vi "Save Local Images Direct.vi"(2 "Save Images":bool, 3 "Image Pathnames":path[](array[path]), 4 "Camera Names":string[](array[string])) -> (0 "error out":errorcluster, 1 "Filenames out":path[](array[path]))   [LabVIEW 2022 SP3]
uses:
  Camera Server/Globals/CamServer global.vi
  Anemometry Sub Vis/Globals/Meas_global.vi
  Anemometry Sub Vis/Globals/Extra_Commands_Global.vi
  Picture Display Global.vi
  Anemometry Sub Vis/Globals/Trav_pos_global.vi
panel:
  out "Execution:State":T1(ring)
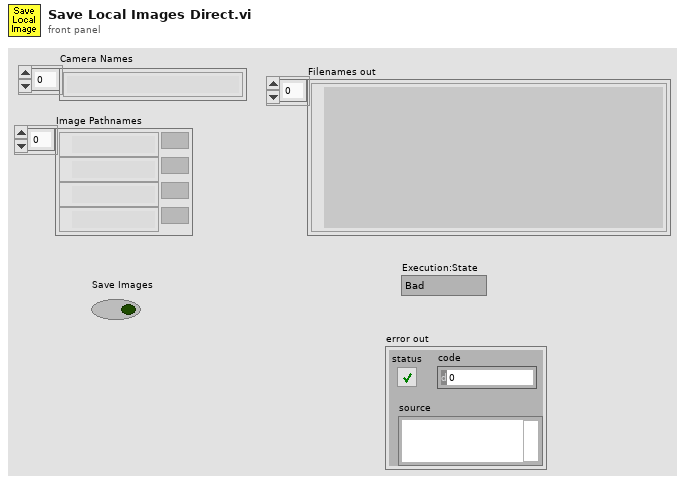
[diagram p1: front panel]
types:
  T1 = enum32{"Bad", "Idle", "Run top level", "Running"}
  T2 = enum32{"Invalid", "Standard", "Closed", "Hidden", "Minimized", "Maximized"}
  T3 = typedef "Camera enum.ctl" = string
  T4 = typedef "IMAQ Image.ctl" = refnum<image>
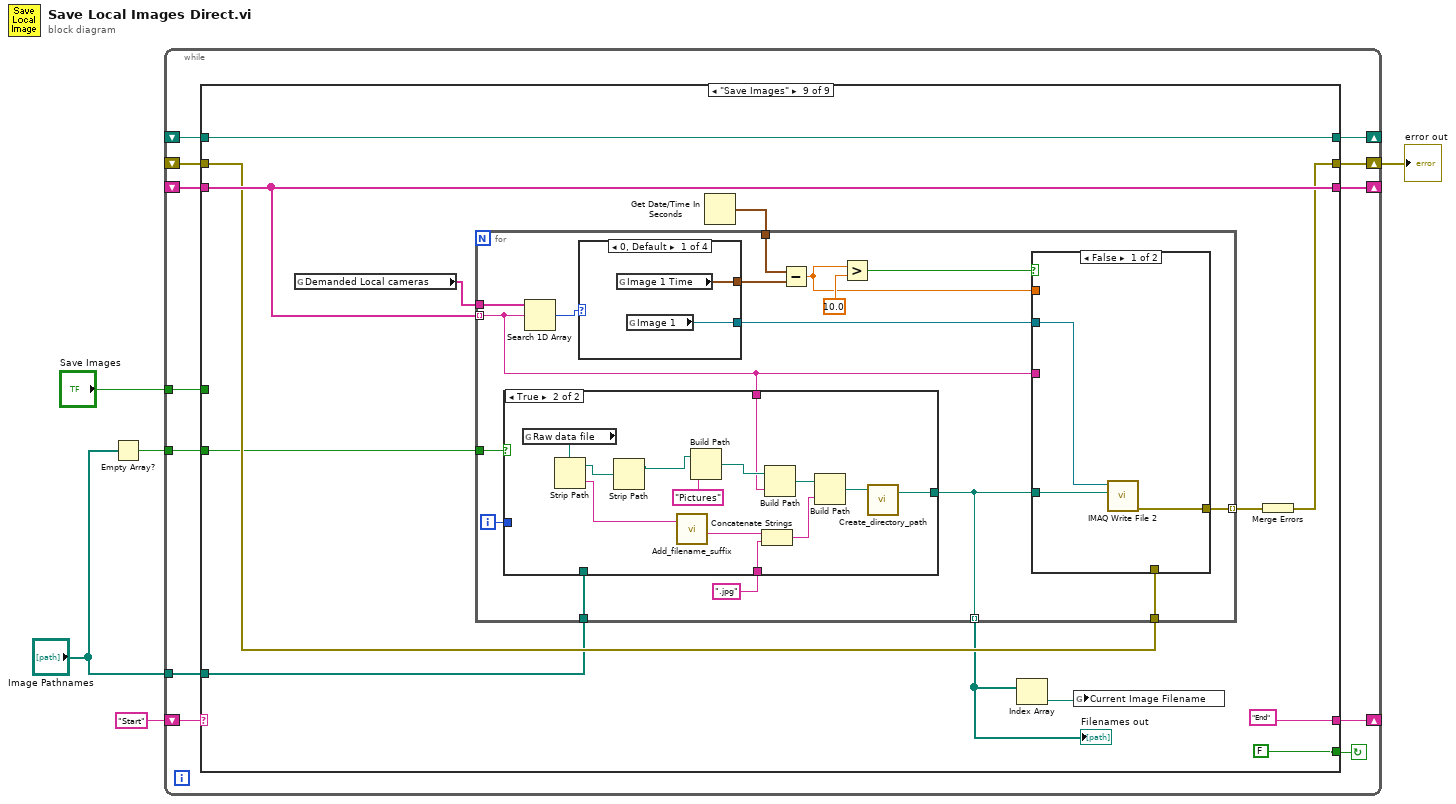
[diagram p0: block diagram]
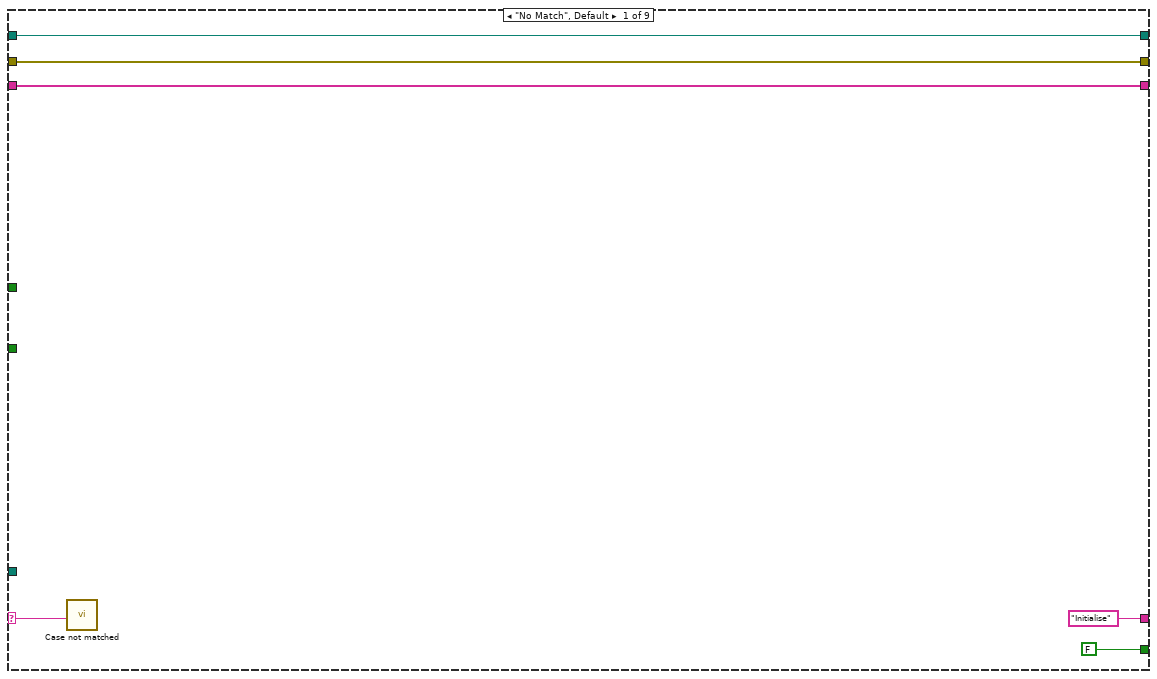
[diagram p2: hidden frame]
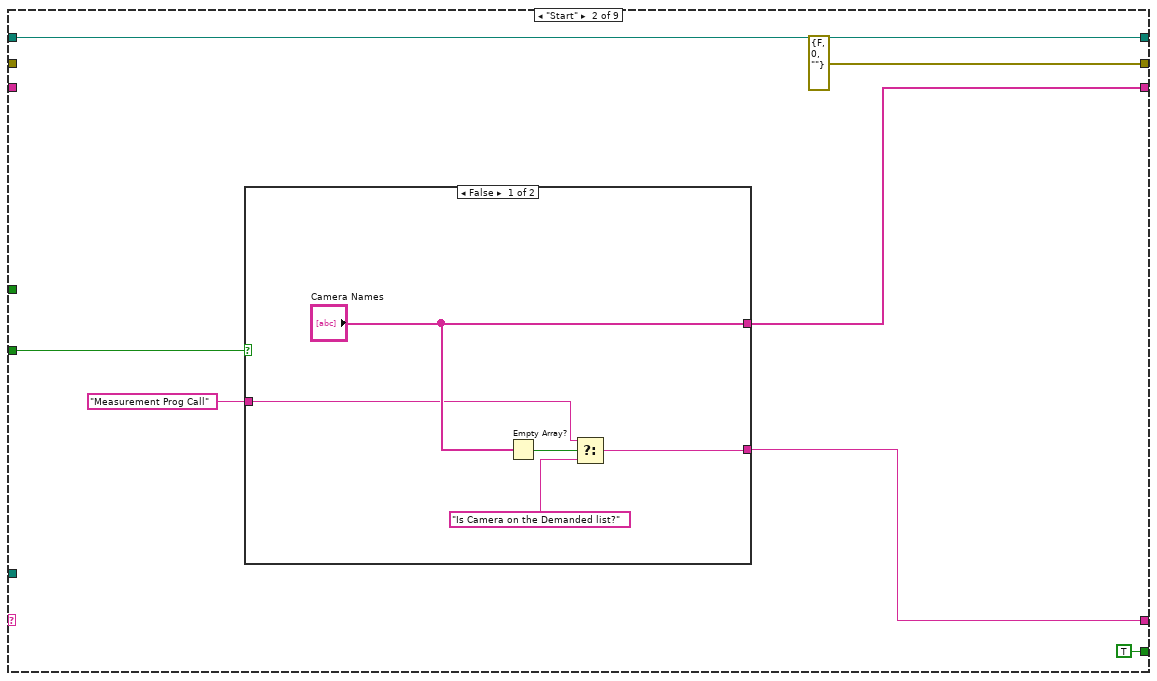
[diagram p3: hidden frame]
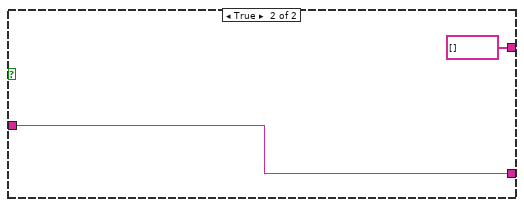
[diagram p4: hidden frame]
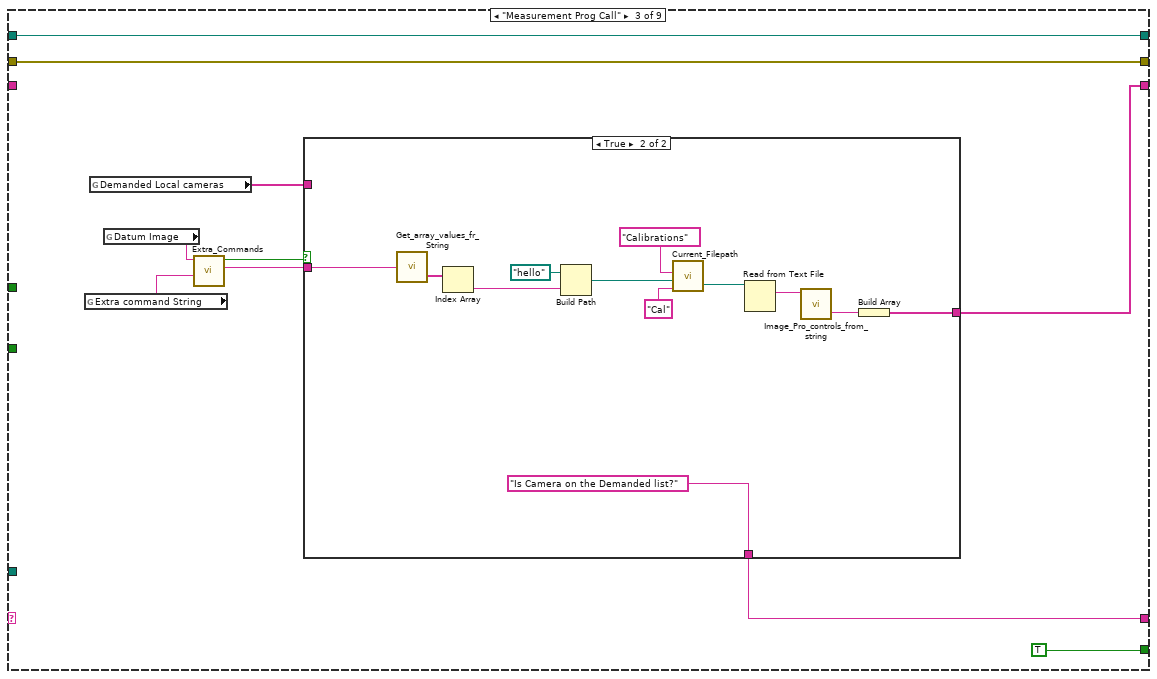
[diagram p5: hidden frame]
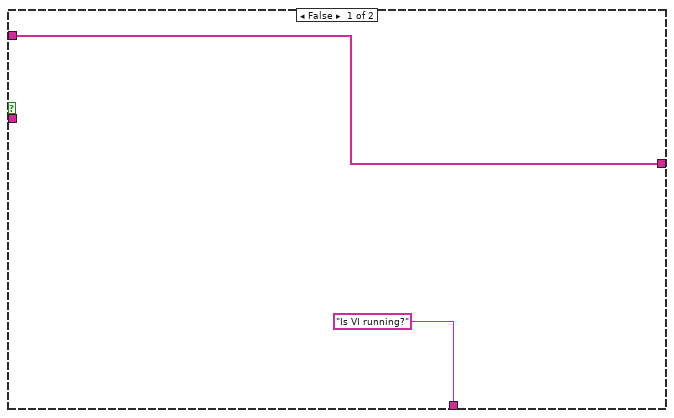
[diagram p6: hidden frame]
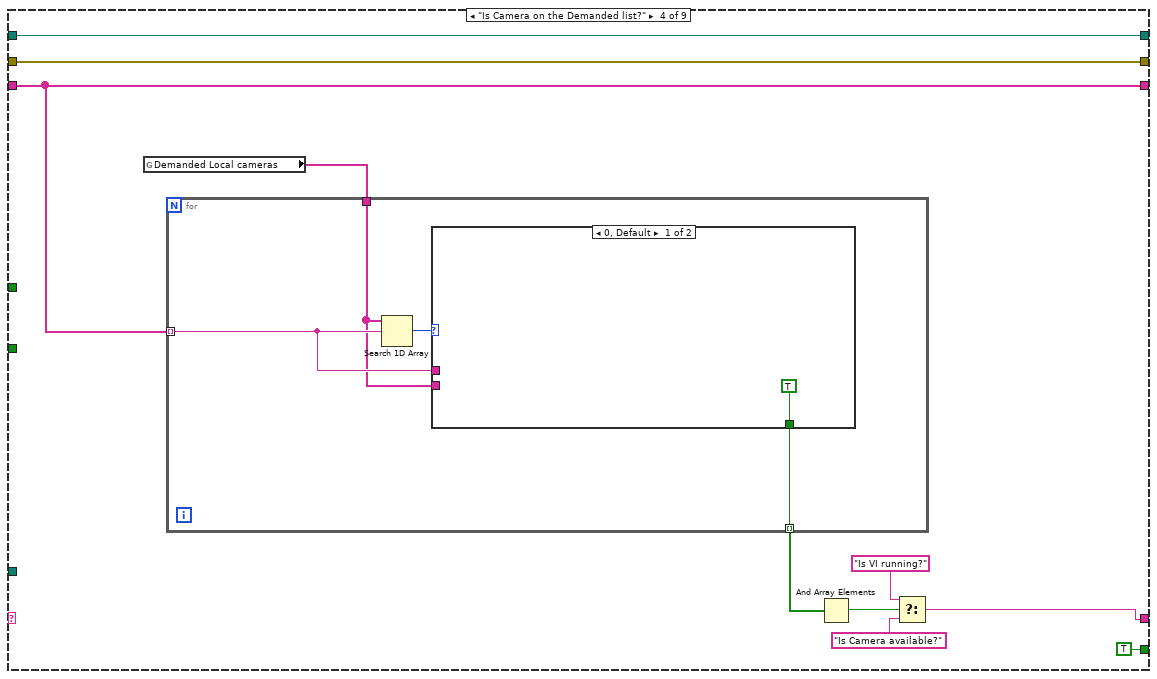
[diagram p7: hidden frame]
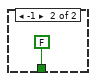
[diagram p8: hidden frame]
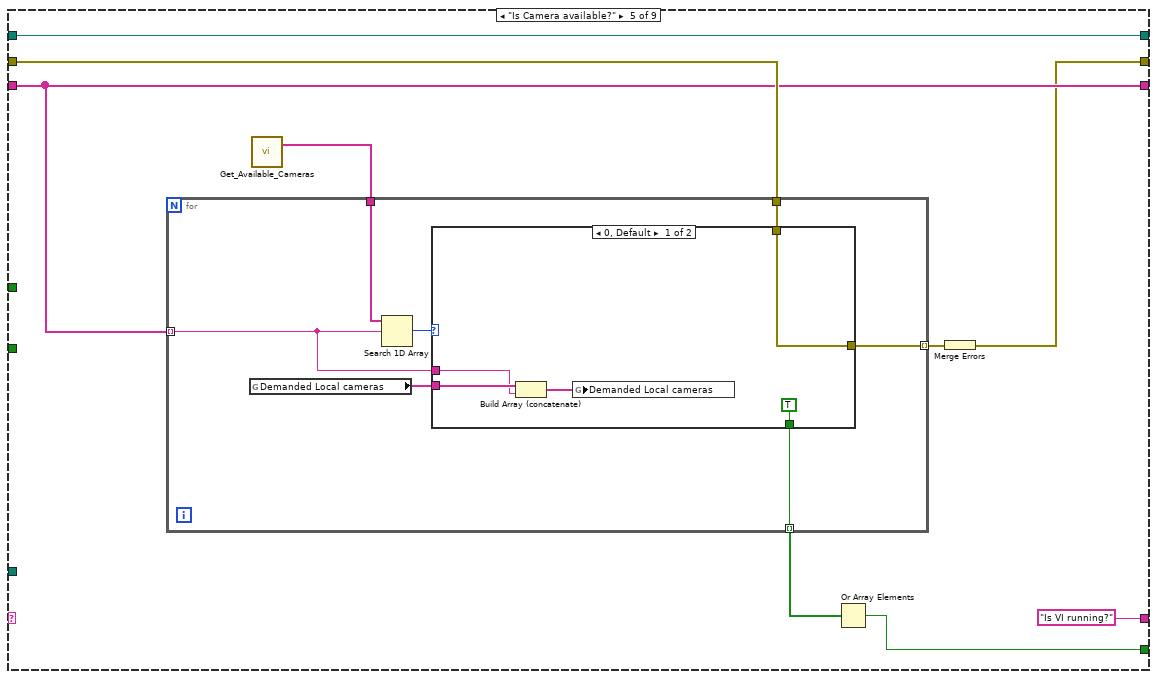
[diagram p9: hidden frame]
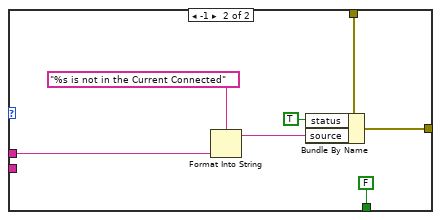
[diagram p10: hidden frame]
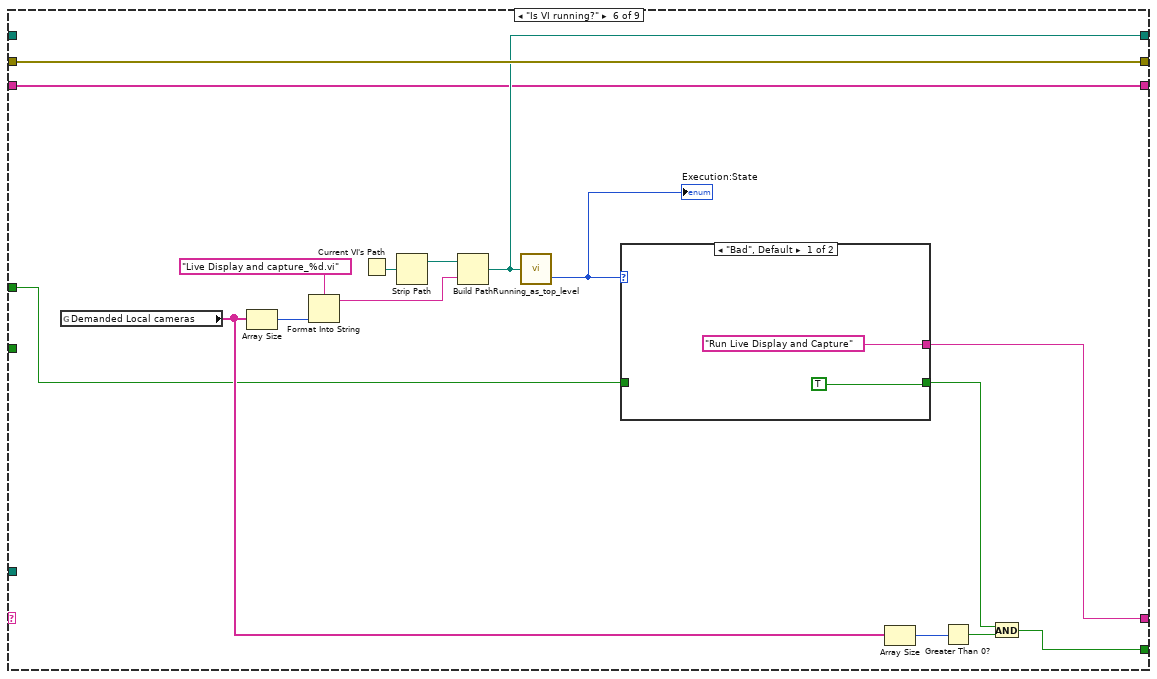
[diagram p11: hidden frame]
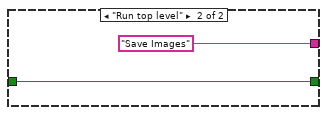
[diagram p12: hidden frame]
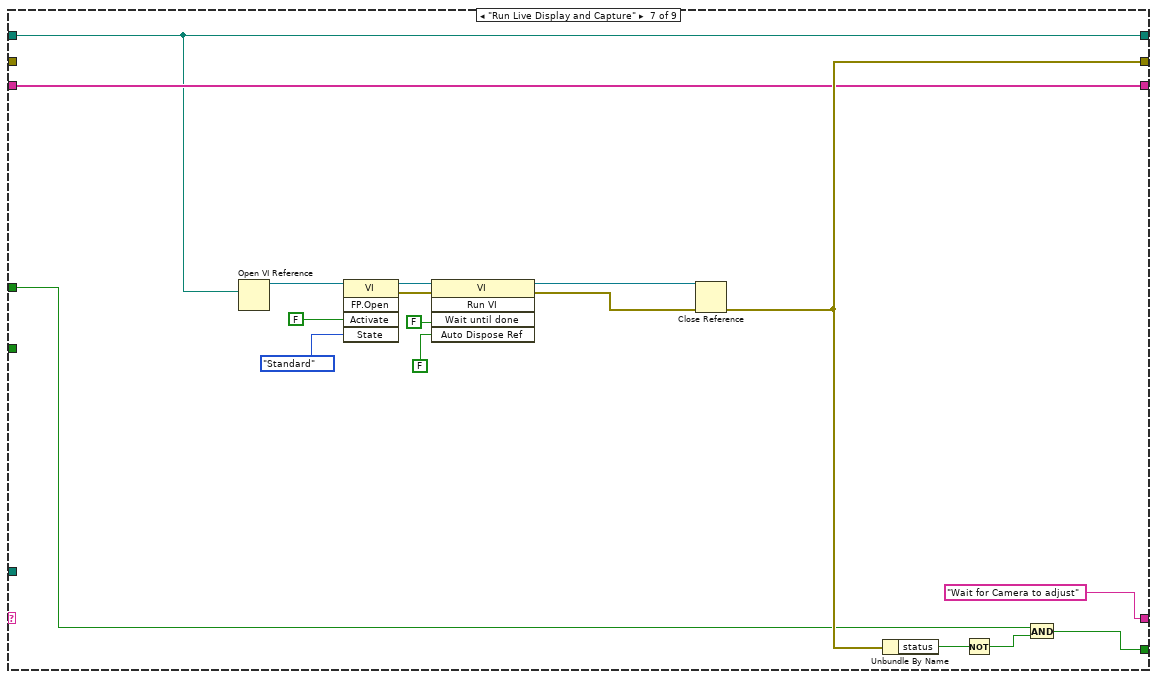
[diagram p13: hidden frame]
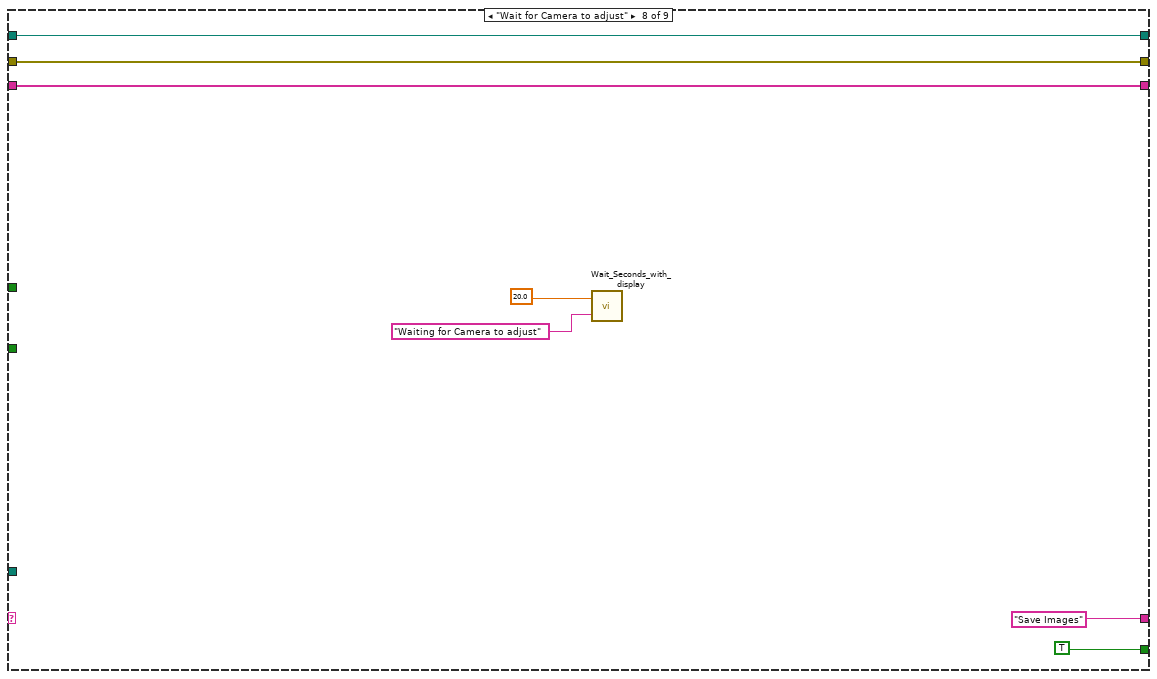
[diagram p14: hidden frame]
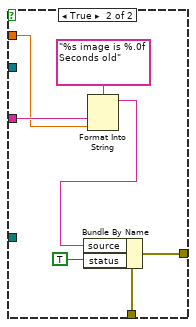
[diagram p15: hidden frame]
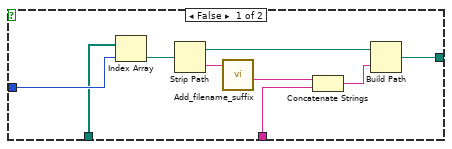
[diagram p16: hidden frame]
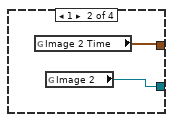
[diagram p17: hidden frame]
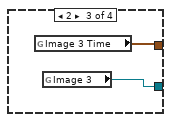
[diagram p18: hidden frame]
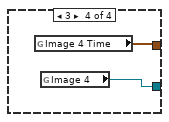
[diagram p19: hidden frame]
diagram:
  n1 = Empty Array?(array="Image Pathnames") -> (empty?=w3:bool)
  n2 = while {
    shift-left: "Start" -> [w15]
    shift-right: [w16] -> _
    shift-right: [w14] -> w4
    shift-left: _ -> [w13]
    shift-right: [w12] -> _
    shift-left: _ -> [w11]
    shift-right: [w10] -> _
    shift-left: _ -> [w9]
    tunnel: w3 -> [w8]
    tunnel: "Image Pathnames" -> [w7]
    tunnel: "Save Images" -> [w6]
    stop <- w17 continue-if-true
    n3 = case shown="\"Save Images\"" w15 {
      selector: w15 -> [w20 _ _ _ _ _ _ _ _]
      tunnel: [FALSE TRUE ("Save Images") TRUE ("Save Images") TRUE ("Save Images") w78 w107 w127 TRUE ("Save Images") FALSE] -> w17
      tunnel: ["Initialise" w26 w39 w63 "Is VI running?" w120 "Wait for Camera to adjust" "Save Images" "End"] -> w16
      tunnel: [w21 errorcluster {"status"=FALSE, "code"=0, "source"=""} ("error out") w38 w67 w80 w119 w133 w145 w158] -> w14
      tunnel: w13 -> [w21 _ w38 w67 w84 w119 _ w145 w154]
      tunnel: [w18 w27 w47 w70 w82 w111 w131 w144 w159] -> w12
      tunnel: w11 -> [w18 _ _ w70 w82 w111 w131 w144 w159]
      tunnel: [w19 w30 w46 w71 w86 w115 w130 w143 w160] -> w10
      tunnel: w9 -> [w19 w30 w46 w71 w86 _ w130 w143 w160]
      tunnel: w8 -> [_ w29 _ _ _ _ _ _ w151]
      tunnel: w7 -> [_ _ _ _ _ _ _ _ w150]
      tunnel: w6 -> [_ _ _ _ _ w106 w126 _ _]
      frame "No Match", Default {
        n4 = call "Case not matched.vi"("Case Name not Matched"=w20) -> ()
      }
      frame "Start" {
        n5 = case shown="False" w29 {
          tunnel: ["Camera Names" string[] [] ("Camera Names")] -> w27
          tunnel: [w32 w36] -> w26
          tunnel: "Measurement Prog Call" -> [w31 w36]
          frame False {
            n6 = Empty Array?(array="Camera Names") -> (empty?=w33:bool)
            n7 = Select(t=w31, s=w33, f="Is Camera on the Demanded list?") -> (s? t:f=w32:string)
          }
          frame True {
          }
        }
      }
      frame "Measurement Prog Call" {
        n8 = global read "Meas_global.vi" "Extra command String"() -> (w44:string)
        n9 = global read "CamServer global.vi" "Demanded Local cameras"() -> (w41:T3[])
        n10 = global read "Extra_Commands_Global.vi" "Datum Image"() -> (w45:string)
        n11 = call "Extra_Commands.vi"("String to Search"=w44, "Command"=w45) -> ("String Value"=w42:string, "Command Found"=w43:bool)  [unwired: 2 in, 2 out]
        n12 = case shown="True" w43 {
          tunnel: [w49 w52] -> w47
          tunnel: w41 -> [w49 _]
          tunnel: w42 -> [_ w56]
          tunnel: ["Is VI running?" "Is Camera on the Demanded list?"] -> w39
          frame False {
          }
          frame True {
            n13 = call "Get_array_values_fr_String.vi"("String Value"=w56) -> ("String array"=w60:string[])  [unwired: 1 out]
            n14 = Index Array(array=w60) -> (element=w61:string)  [unwired: 1 in]
            n15 = Build Path(base path=path "hello", name or relative path=w61) -> (appended path=w58:path)
            n16 = call "Current_Filepath.vi"("Short_Name"="Cal" ("Data Type"), "Filename in"=w58, "Data Type"="Calibrations") -> ("Filename Out"=w57:path)  [unwired: 1 in, 1 out]
            n17 = Read from Text File(file (use dialog)=w57) -> (text=w59:string)  [unwired: 3 in, 3 out]
            n18 = call "Image_Pro_controls_from_string.vi"("Setup String"=w59) -> ("Camera"=w51:string)  [unwired: 6 in, 4 out]
            n19 = Build Array(w51) -> (w52:string[])
          }
        }
      }
      frame "Is Camera on the Demanded list?" {
        n20 = global read "CamServer global.vi" "Demanded Local cameras"() -> (w68:T3[])
        n21 = for {
          tunnel: w68 -> [w72]
          tunnel: w70 -> [w74] mode=indexing
          tunnel: [w73] -> w69 mode=indexing
          n22 = Search 1D Array(1D array=w72, element=w74) -> (index of element=w75:i32)  [unwired: 1 in]
          n23 = case shown="0, Default" w75 {
            tunnel: w74 -> [_ _]
            tunnel: w72 -> [_ _]
            tunnel: [TRUE ("Save Images") FALSE ("Save Images")] -> w73
            frame 0, Default {
            }
            frame -1 {
            }
          }
        }
        n24 = And Array Elements(Boolean array=w69) -> (logical AND=w64:bool)
        n25 = Select(t="Is VI running?", s=w64, f="Is Camera available?") -> (s? t:f=w63:string)
      }
      frame "Is Camera available?" {
        n26 = call "Get_Available_Cameras.vi"() -> ("Cameras"=w85:string[])  [unwired: 2 in, 1 out]
        n27 = for {
          tunnel: w85 -> [w93]
          tunnel: w82 -> [w91] mode=indexing
          tunnel: w84 -> [w89]
          tunnel: [w88] -> w81 mode=indexing
          tunnel: [w87] -> w79 mode=indexing
          n28 = global read "CamServer global.vi" "Demanded Local cameras"() -> (w90:T3[])
          n29 = Search 1D Array(1D array=w93, element=w91) -> (index of element=w92:i32)  [unwired: 1 in]
          n30 = case shown="0, Default" w92 {
            tunnel: w91 -> [w96 w102]
            tunnel: w90 -> [w98 _]
            tunnel: w89 -> [w94 w101]
            tunnel: [w94 w100] -> w88
            tunnel: [TRUE ("Save Images") FALSE ("Save Images")] -> w87
            frame 0, Default {
              n31 = Build Array (concatenate)(w98, w96) -> (w97:T3[])
              n32 = global write "CamServer global.vi" "Demanded Local cameras"(w97) -> ()
            }
            frame -1 {
              n33 = Format Into String(format string="%s is not in the Current Connected", w102) -> (resulting string=w104:string)  [unwired: 2 in, 1 out]
              n34 = Bundle By Name(cluster=w101, "status"=TRUE, "source"=w104) -> (w100:errorcluster)
            }
          }
        }
        n35 = Or Array Elements(Boolean array=w79) -> (logical OR=w78:bool)
        n36 = Merge Errors(w81) -> (w80:errorcluster)
      }
      frame "Is VI running?" {
        n37 = global read "CamServer global.vi" "Demanded Local cameras"() -> (w110:T3[])
        n38 = Array Size(array=w110) -> (size(s)=w116:i32)
        n39 = Format Into String(format string="Live Display and capture_%d.vi", w116) -> (resulting string=w118:string)  [unwired: 2 in, 1 out]
        n40 = Current VI's Path() -> (path=w114:path)
        n41 = Strip Path(path=w114) -> (stripped path=w113:path)  [unwired: 1 out]
        n42 = Build Path(base path=w113, name or relative path=w118) -> (appended path=w115:path)
        n43 = call "Running_as_top_level.vi"("Vi path name"=w115) -> ("Execution:State"=w121:T1)  [unwired: 1 out]
        "Execution:State" <- w121
        n44 = case shown="\"Bad\", Default" w121 {
          tunnel: ["Run Live Display and Capture" "Save Images"] -> w120
          tunnel: [TRUE w124] -> w108
          tunnel: w106 -> [_ w124]
          frame "Bad", Default {
          }
          frame "Run top level" {
          }
        }
        n45 = Array Size(array=w110) -> (size(s)=w112:i32)
        n46 = Greater Than 0?(x=w112) -> (x > 0?=w109:bool)
        n47 = And(x=w108, y=w109) -> (x .and. y?=w107:bool)
      }
      frame "Run Live Display and Capture" {
        n48 = Open VI Reference(vi path=w130) -> (vi reference=w142:refnum<vi>)  [unwired: 3 in, 3 out]
        n49 = invoke class="VI" method="FP.Open"(reference=w142, "Activate"=FALSE ("Activate?"), "State"=T2."Standard") -> (reference out=w139:refnum<vi>, error out=w138:errorcluster)  [unwired: 2 in, 3 out]
        n50 = invoke class="VI" method="Run VI"(reference=w139, error in=w138, "Wait until done"=FALSE ("Wait Until Done"), "Auto Dispose Ref"=FALSE ("Auto Dispose Reference")) -> (reference out=w137:refnum<vi>, error out=w136:errorcluster)  [unwired: 1 in, 3 out]
        n51 = Close Reference(reference=w137, error in (no error)=w136) -> (error out=w133:errorcluster)
        n52 = Unbundle By Name(w133) -> ("status"=w132:bool)
        n53 = Not(x=w132) -> (.not. x?=w128:bool)
        n54 = And(x=w126, y=w128) -> (x .and. y?=w127:bool)
      }
      frame "Wait for Camera to adjust" {
        n55 = call "Wait_Seconds_with_display.vi"("Message"="Waiting for Camera to adjust", "Seconds to wait"=20.0) -> ()  [unwired: 1 in, 1 out]
      }
      frame "Save Images" {
        n56 = global read "CamServer global.vi" "Demanded Local cameras"() -> (w157:T3[])
        n57 = Get Date/Time In Seconds() -> (seconds since 1Jan1904=w156:timestamp)
        n58 = for {
          tunnel: w159 -> [w171] mode=indexing
          tunnel: w157 -> [w178]
          tunnel: w150 -> [w176]
          tunnel: w156 -> [w173]
          tunnel: [w169] -> w155 mode=indexing
          tunnel: w154 -> [w166]
          tunnel: [w165] -> w153 mode=indexing
          tunnel: w151 -> [w164]
          i -> [w175]
          n59 = case shown="True" w164 {
            tunnel: w171 -> [_ w202]
            tunnel: [w190 w201] -> w165
            tunnel: w176 -> [w196 _]
            tunnel: w175 -> [w197 _]
            tunnel: ".jpg" ("string") -> [w189 w200]
            frame False {
              n60 = Index Array(array=w196, index=w197) -> (element=w194:path)
              n61 = Strip Path(path=w194) -> (stripped path=w191:path, name=w193:string)
              n62 = call "Add_filename_suffix.vi"("Filename"=w193) -> ("Base name"=w195:string)  [unwired: 1 in, 3 out]
              n63 = Concatenate Strings(w195, w189) -> (w192:string)
              n64 = Build Path(base path=w191, name or relative path=w192) -> (appended path=w190:path)
            }
            frame True {
              n65 = global read "Meas_global.vi" "Raw data file"() -> (w207:path)
              n66 = Strip Path(path=w207) -> (stripped path=w199:path, name=w206:string)
              n67 = Strip Path(path=w199) -> (stripped path=w198:path)  [unwired: 1 out]
              n68 = call "Add_filename_suffix.vi"("Filename"=w206) -> ("Base name"=w209:string)  [unwired: 1 in, 3 out]
              n69 = Build Path(base path=w198, name or relative path="Pictures") -> (appended path=w208:path)
              n70 = Concatenate Strings(w209, w200) -> (w204:string)
              n71 = Build Path(base path=w208, name or relative path=w202) -> (appended path=w205:path)
              n72 = Build Path(base path=w205, name or relative path=w204) -> (appended path=w203:path)
              n73 = call "Create_directory_path.vi"("Path name"=w203) -> ("Path name Out"=w201:path)  [unwired: 2 in, 1 out]
            }
          }
          n74 = Search 1D Array(1D array=w178, element=w171) -> (index of element=w177:i32)  [unwired: 1 in]
          n75 = case shown="0, Default" w177 {
            tunnel: [w212 w214 w216 w218] -> w167
            tunnel: [w211 w213 w215 w217] -> w174
            frame 0, Default {
              n76 = global read "Picture Display Global.vi" "Image 1 Time"() -> (w211:timestamp)
              n77 = global read "Picture Display Global.vi" "Image 1"() -> (w212:T4)
            }
            frame 1 {
              n78 = global read "Picture Display Global.vi" "Image 2 Time"() -> (w213:timestamp)
              n79 = global read "Picture Display Global.vi" "Image 2"() -> (w214:T4)
            }
            frame 2 {
              n80 = global read "Picture Display Global.vi" "Image 3 Time"() -> (w215:timestamp)
              n81 = global read "Picture Display Global.vi" "Image 3"() -> (w216:T4)
            }
            frame 3 {
              n82 = global read "Picture Display Global.vi" "Image 4 Time"() -> (w217:timestamp)
              n83 = global read "Picture Display Global.vi" "Image 4"() -> (w218:T4)
            }
          }
          n84 = Subtract(x=w173, y=w174) -> (x-y=w170:dbl)
          n85 = Greater?(x=w170, y=10.0) -> (0:w168:bool)
          n86 = case shown="False" w168 {
            tunnel: w171 -> [_ w188]
            tunnel: w170 -> [_ w187]
            tunnel: [w179 w186] -> w169
            tunnel: w165 -> [w181 _]
            tunnel: w167 -> [w180 _]
            tunnel: w166 -> [_ w182]
            frame False {
              n87 = call-poly "IMAQ Write File 2"("File Path"=w181, "Image"=w180) -> ("error out"=w179:errorcluster)  [unwired: 8 in, 1 out]
            }
            frame True {
              n88 = Format Into String(format string="%s image is %.0f Seconds old", w188, w187) -> (resulting string=w183:string)  [unwired: 2 in, 1 out]
              n89 = Bundle By Name(cluster=w182, "source"=w183, "status"=TRUE) -> (w186:errorcluster)
            }
          }
        }
        "Filenames out" <- w153
        n90 = Index Array(array=w153) -> (element=w152:path)  [unwired: 1 in]
        n91 = global write "Trav_pos_global.vi" "Current Image Filename"(w152) -> ()
        n92 = Merge Errors(w155) -> (w158:errorcluster)
      }
    }
  }
  "error out" <- w4
